vi "MAIN_save_XY_positions.vi"(5 "queue ASI stage":refnum<queue>, 6 "XY positions":refnum<vi>, 7 "XY positions":dbl[][](array[numeric]), 8 "error in":errorcluster, 9 "Start acquisition":bool, 10 "ROI manager":i32(listbox), 11 "ROI manager":refnum<vi>) -> (0 "error out":errorcluster, 2 "Next task":T1, 3 "XY positions OUT":dbl[][](array[numeric]), 4 "XY graph":cluster{dbl[], dbl[]}[](array[cluster]))   [LabVIEW 2015]
uses:
  CONTROLS/Q_ASI_stage_element.ctl
  CONTROLS/Q_main_element.ctl
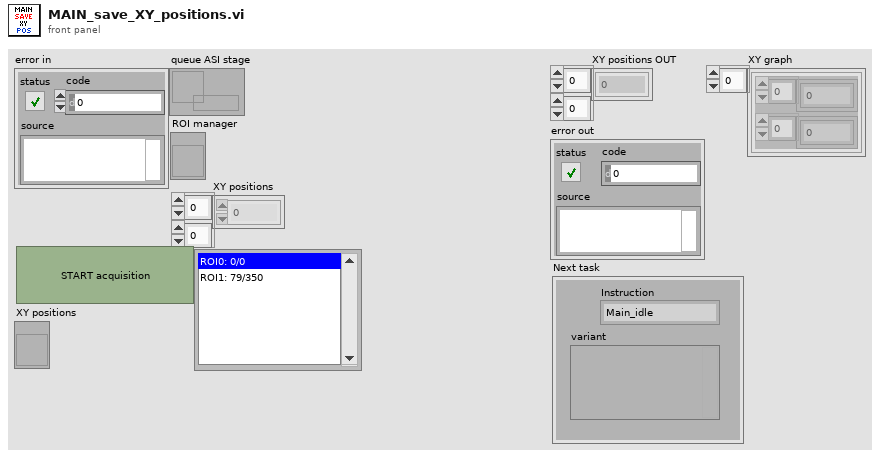
[diagram p1: front panel]
types:
  T1 = typedef "Q_main_element.ctl" = cluster{"variant":variant, "Instruction":enum16{"Main_idle", "Main_initialize", "Main_initialize_TDMS", "Main_initialize_Queue", "Main_error", "Main_DAQ_initialization_results", "Main_ASI_initialization_results", "Main_Piezo_initialization_results", "Main_Valve_initialization_results", "Main_Pump_initialization_results", "Main_CAMERA_initialization_results", "Main_FPGA_initialization_results", "Main_DAQ_error", "Main_ASI_error", "Main_Piezo_error", "Main_CAMERA_error", "Main_Valve_error", "Main_Pump_error", "Main_FPGA_error", "Main_start_acquiring", "Main_not_acquiring", "Main_acquiring", "Main_stop_acquiring", "Main_change_exposure", "Main_change_z_scan_parameters", "Main_define_ROI", "Main_define_mosaic", "Main_read_kinetic_time", "Main_cooler", "Main_read_temperature", "Main_save_XY", "Main_load_XY", "Main_discard_XY", "Main_move_to_XY", "Main_measure_QPD", "Main_autofocus_calibration", "Main_autofocus_initialization", "Main_autofocus_stop", "Main_save_PID", "Main_change_H_valve_position", "Main_two_way_valve", "Main_save_movie", "Main_init_single_scan", "Main_single_scan", "Main_stop_single_scan", "Main_merFISH_illumination_parameters", "Main_merFISH_buffer_probe_list", "Main_merFISH_injections_procedure", "Main_merFISH_save_setpoint", "Main_merFISH_DAPI_parameters", "Main_merFISH_Brightfield_parameters", "Main_merFISH_save_embryo_ROI", "Main_merFISH_init", "Main_merFISH_resume", "Main_merFISH_start_autofocus", "Main_merFISH_open_close_valve_merFISH", "Main_merFISH_open_close_valve_photobleaching", "Main_merFISH_hybridization", "Main_merFISH_move_to_ROI", "Main_merFISH_wait_stabilization", "Main_merFISH_move_to_REF", "Main_merFISH_scan", "Main_merFISH_photobleaching_injection", "Main_merFISH_photobleaching", "Main_merFISH_send_email", "Main_merFISH_close", "Main_STOP"}}
  T2 = typedef "Q_ASI_stage_element.ctl" = cluster{"variant":variant, "Instruction":enum16{"ASI_idle", "ASI_initialize", "ASI_error", "ASI_security_stop", "ASI_read_XYZ", "ASI_up", "ASI_down", "ASI_left", "ASI_right", "ASI_save_XY", "ASI_move_to_XY", "ASI_brightfield", "ASI_init_scan", "ASI_init_merFISH", "ASI_move_to_XY_merFISH", "ASI_move_to_Z_merFISH", "ASI_init_autofocus_search_merFISH", "ASI_close_autofocus_search_merFISH", "ASI_adjust_piezo_autofocus_merFISH", "ASI_set_piezo_autofocus_to_reference_position_merFISH_TL", "ASI_close_merFISH", "ASI_stop"}}
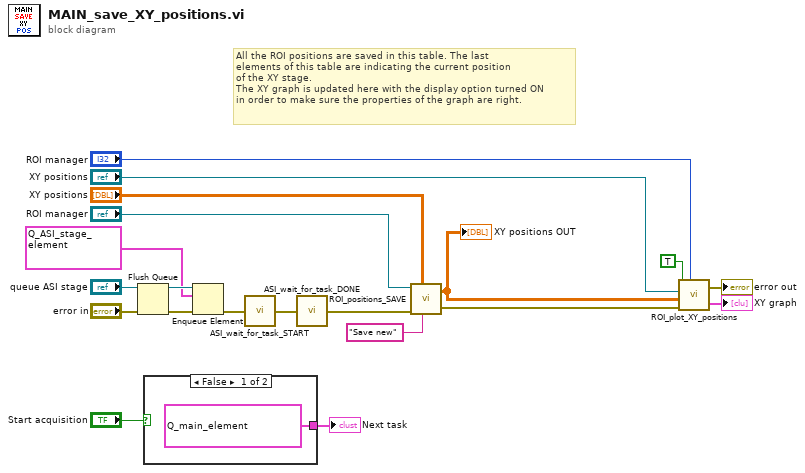
[diagram p0: block diagram]
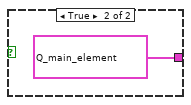
[diagram p2: hidden frame]
diagram:
  # "All the ROI positions are saved in this table. The last \nelements of this table are indicating the current position\nof the XY stage.\nThe XY graph is updated here with the display option turned ON\nin order to make sure the properties of the graph are right."
  n1 = Flush Queue(queue="queue ASI stage", error in (no error)="error in") -> (queue out=w12:refnum<queue>, error out=w13:errorcluster)  [unwired: 1 out]
  n2 = case shown="False" "Start acquisition" {
    tunnel: [T1 {"variant"=variant, "Instruction"=enum."Main_not_acquiring"} ("Q_main_element") T1 {"variant"=variant, "Instruction"=enum."Main_acquiring"} ("Q_main_element")] -> w1
    frame False {
    }
    frame True {
    }
  }
  "Next task" <- w1
  n3 = Enqueue Element(queue=w12, element=T2 {"variant"=variant, "Instruction"=enum."ASI_save_XY"} ("Q_ASI_stage"), error in (no error)=w13) -> (error out=w14:errorcluster)  [unwired: 1 in, 2 out]
  n4 = call "ASI_wait_for_task_START.vi"("error in"=w14) -> ("error out"=w15:errorcluster)
  n5 = call "ASI_wait_for_task_DONE.vi"("error in"=w15) -> ("error out"=w17:errorcluster)
  n6 = call "ROI_positions_SAVE.vi"("Choice"="Save new", "XY positions"="XY positions", "error in"=w17, "ROI LstBox Refnum"="ROI manager") -> ("error out"=w19:errorcluster, "XY positions OUT"=w20:dbl[][])  [unwired: 2 in]
  "XY positions OUT" <- w20
  n7 = call "ROI_plot_XY_positions.vi"("Display?"=TRUE, "XYGraph Refnum"="XY positions", "XY positions"=w20, "error in"=w19, "ROI manager"="ROI manager") -> ("error out"=→"error out":errorcluster, "XY graph"=→"XY graph":cluster{dbl[], dbl[]}[])
